vi "Batch Offset Retrieval.vi"(7 "Tag":string, 8 "error in":errorcluster, 11 "Transactions":T1[](array[typedef])) -> (0 "error out":errorcluster, 3 "Data":dbl[][](array[numeric]))   [LabVIEW 2009]
uses:
  Global Data/Transactions/Dataset Transaction Id.ctl
  Global Data/Transactions/Dataset Source.ctl
  Global Data/Transactions/Dataset Type.ctl
  Apps/Yes No Button.ctl
  Data Access Objects/Metadata/DAO Actions.ctl
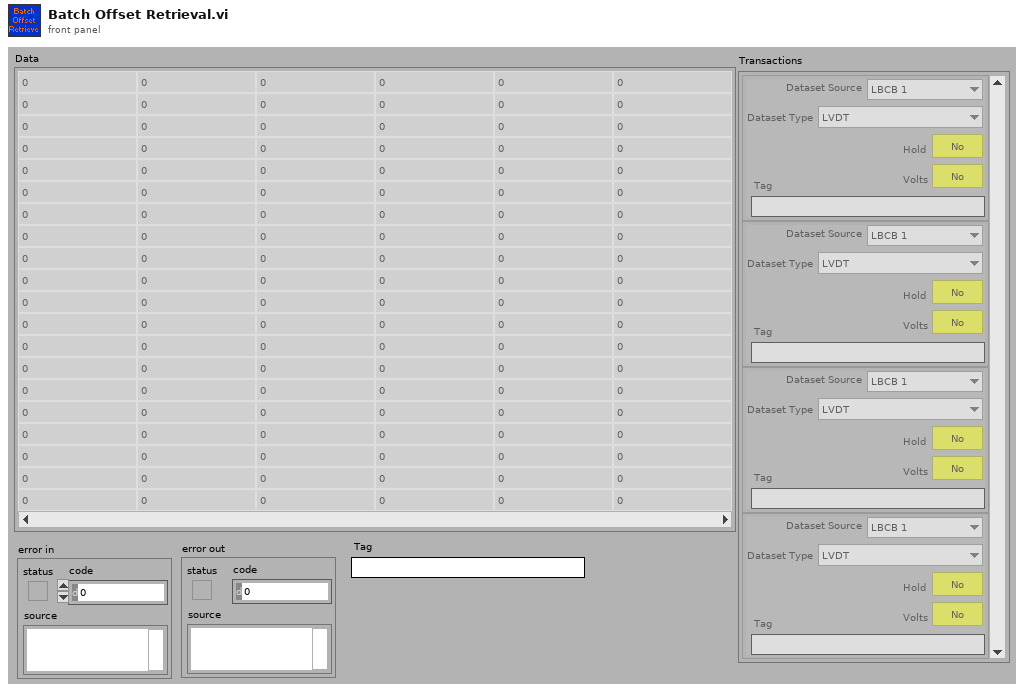
[diagram p1: front panel]
types:
  T1 = typedef "Dataset Transaction Id.ctl" = cluster{"Dataset Source":T2, "Dataset Type":T3, "Hold":T4, "Volts":T4, "Tag":string}
  T2 = typedef "Dataset Source.ctl" = enum16{"LBCB 1", "LBCB 2", "Combined", "External Sensors"}
  T3 = typedef "Dataset Type.ctl" = enum16{"LVDT", "Load Cell", "Actuator Command", "Servo Error", "Displacement Command", "Displacement", "Force"}
  T4 = typedef "Yes No Button.ctl" = bool
  T5 = typedef "DAO Actions.ctl" = enum16{"Init", "Get", "Set"}
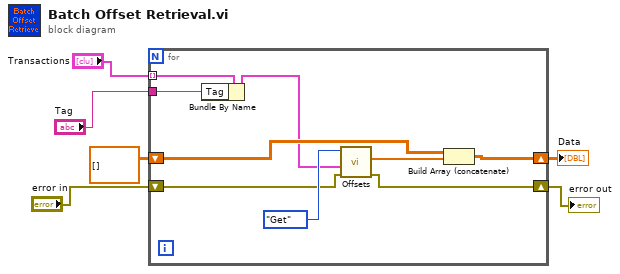
[diagram p0: block diagram]
diagram:
  n1 = for {
    shift-right: [w13] -> w3
    shift-left: "error in" -> [w12]
    tunnel: "Transactions" -> [w11] mode=indexing
    shift-right: [w10] -> w5
    shift-left: dbl[][] [] -> [w9]
    tunnel: "Tag" -> [w7]
    n2 = Bundle By Name(cluster=w11, "Tag"=w7) -> (w8:T1)
    n3 = call "Offsets.vi"("error in (no error)"=w12, "Dataset Trans Id"=w8, "DAO Actions"=DAO_Actions."Get") -> ("error out"=w13:errorcluster, "Data Out"=w15:dbl[])  [unwired: 6 in, 1 out]
    n4 = Build Array (concatenate)(w9, w15) -> (w10:dbl[][])
  }
  "Data" <- w5
  "error out" <- w3
